vi "Initialize Instrument.vi"(8 "error in (no error)":errorcluster, 10 "Reset":bool, 11 "PSG-MXG in":refnum<class "PSG-MXG.lvclass">) -> (0 "error out":errorcluster, 3 "PSG-MXG out":refnum<class "PSG-MXG.lvclass">)   [LabVIEW 2020, in "PSG-MXG.lvclass"]
uses:
  PSG-MXG.lvclass
  C:/Sandbox/RF Bench/Source Code/WiSpry Test Framework/Instruments/Instrument.lvclass
  Instrument.lvclass/Instrument.ctl
  Instrument.lvclass
  <instrlib>/Agilent PSG MXG Series/Agilent PSG MXG Series.lvlib
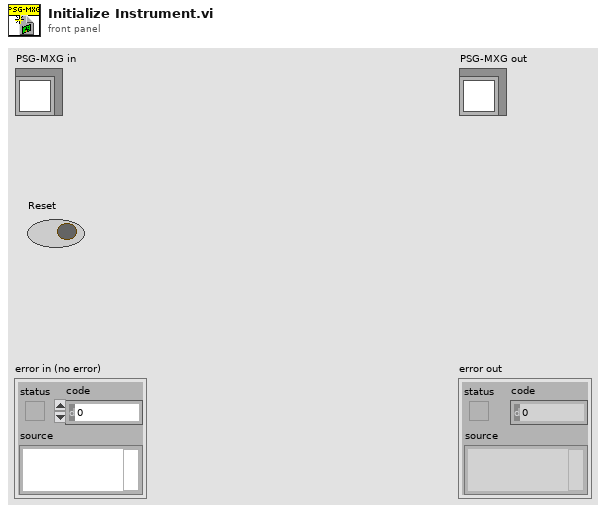
[diagram p1: front panel]
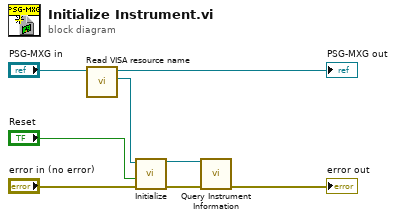
[diagram p0: block diagram]
diagram:
  n1 = call "Read VISA resource name.vi"("Instrument in"="PSG-MXG in") -> ("VISA resource name"=w4:refnum<visa-resource-name>, "Instrument out"=→"PSG-MXG out":refnum<class "PSG-MXG.lvclass">)  [unwired: 9 in]
  n2 = call <instrlib>:"Initialize.vi"("error in (no error)"="error in (no error)", "Reset (True)"="Reset", "VISA resource name"=w4) -> ("error out"=w3:errorcluster, "VISA resource name out"=w1:refnum<visa-resource-name>)  [unwired: 7 in]
  n3 = call <instrlib>:"Query Instrument Information.vi"("VISA resource name"=w1, "error in (no error)"=w3) -> ("error out"=→"error out":errorcluster)  [unwired: 6 in, 7 out]
